vi "Disable FP.vi"(7 "Ignore?":bool, 8 "error in (no error)":errorcluster, 11 "FP Controls in":refnum<class "FP Controls.lvclass">) -> (0 "error out":errorcluster, 3 "FP Controls out":refnum<class "FP Controls.lvclass">)   [LabVIEW 2018, in "Configuration Grandmaster.lvlib" / "FP Controls.lvclass"]
uses:
  FP Controls.lvclass
  FP Controls.lvclass/FP Controls.ctl
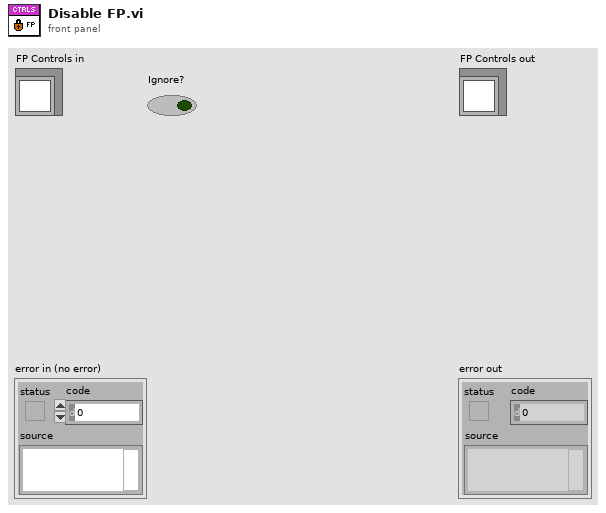
[diagram p1: front panel]
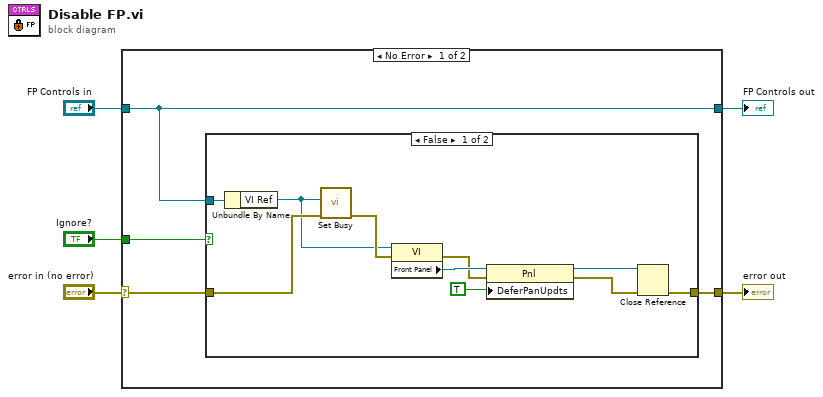
[diagram p0: block diagram]
diagram:
  n1 = case shown="No Error" "error in (no error)" {
    selector: "error in (no error)" -> [w8 w22]
    tunnel: [w7 w22] -> w4
    tunnel: [w9 w21] -> w2
    tunnel: "FP Controls in" -> [w9 w21]
    tunnel: "Ignore?" -> [w6 _]
    frame No Error {
      n2 = case shown="False" w6 {
        tunnel: w9 -> [w19 _]
        tunnel: w8 -> [w18 w20]
        tunnel: [w12 w20] -> w7
        frame False {
          n3 = Unbundle By Name(w19) -> ("VI Ref"=w10:refnum<vi>)
          n4 = call <vilib>:"Set Busy.vi"("error in (no error)"=w18, "VI reference (current VI)"=w10) -> ("error out"=w11:errorcluster)  [unwired: 8 in, 1 out]
          n5 = property class="VI"(reference=w10, error in=w11) -> (error out=w14:errorcluster, "Front Panel"=w17:refnum<vi>)  [unwired: 1 out]
          n6 = property class="Pnl"(reference=w17, error in=w14, "DeferPanUpdts"=TRUE ("Defer Panel Updates")) -> (reference out=w16:refnum<vi>, error out=w15:errorcluster)
          n7 = Close Reference(reference=w16, error in (no error)=w15) -> (error out=w12:errorcluster)
        }
        frame True {
        }
      }
    }
    frame Error {
    }
  }
  "error out" <- w4
  "FP Controls out" <- w2
